vi "新增控件ID.vi"(8 "error in (no error)":errorcluster caption="错误输入（无错误）", 10 "控件ID":u32, 11 "程序响应 输入":refnum<class "程序响应.lvclass">) -> (0 "error out":errorcluster caption="错误输出", 3 "程序响应 输出":refnum<class "程序响应.lvclass">)   [LabVIEW 2018, in "程序响应.lvlib" / "程序响应.lvclass"]
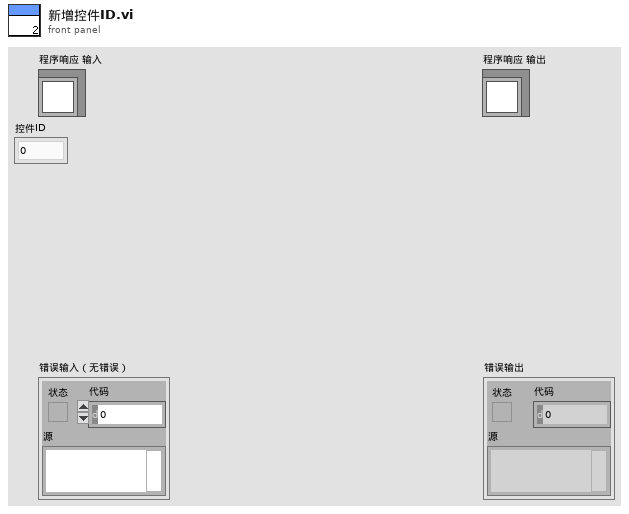
[diagram p1: front panel]
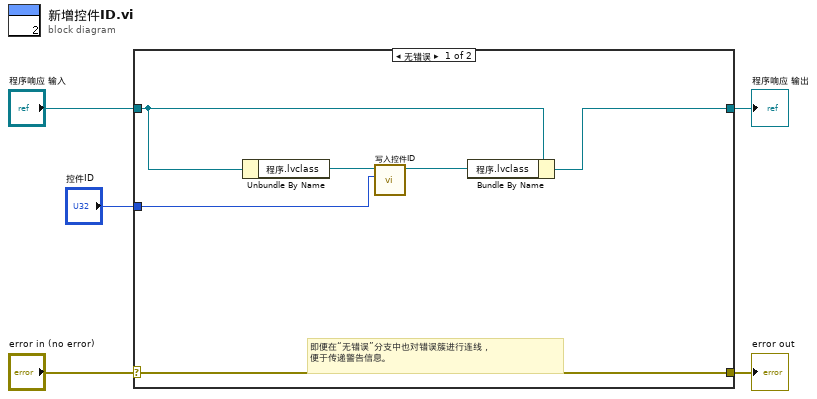
[diagram p0: block diagram]
diagram:
  n1 = case shown="无错误" "error in (no error)" {
    selector: "error in (no error)" -> [w11 w13]
    tunnel: [w11 w13] -> w4
    tunnel: [w7 w12] -> w2
    tunnel: "程序响应 输入" -> [w8 w12]
    tunnel: "控件ID" -> [w6 _]
    frame No Error {
      # "即便在“无错误”分支中也对错误簇进行连线，\n便于传递警告信息。"
      n2 = Unbundle By Name(w8) -> ("程序.lvclass"=w10:refnum<class "程序.lvclass">)
      n3 = call-dynamic "写入控件ID.vi"("控件ID"=w6, "程序输入"=w10) -> ("程序输出"=w9:refnum<class "程序.lvclass">)  [unwired: 8 in, 1 out]
      n4 = Bundle By Name(cluster=w8, "程序.lvclass"=w9) -> (w7:refnum<class "程序响应.lvclass">)
    }
    frame Error {
    }
  }
  "error out" <- w4
  "程序响应 输出" <- w2
